vi "getSinglePathElement.vi"(8 "error in (no error)":errorcluster, 9 "Variant in":variant, 10 "JSON String":string, 11 "String":string) -> (0 "error out":errorcluster, 3 "Variant out":variant)   [LabVIEW 2015, in "Zen Analytics.lvclass"]
uses:
  Zen Analytics.lvclass
  <vilib>/addons/_JKI.lib/Serialization/JSON/JKI JSON Serialization.lvlib
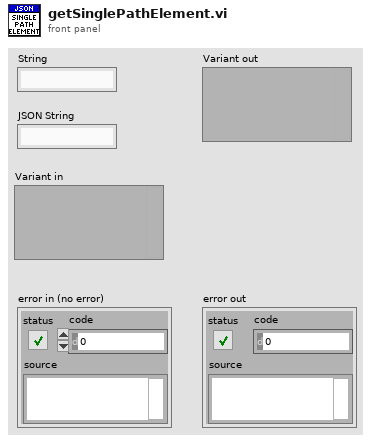
[diagram p1: front panel]
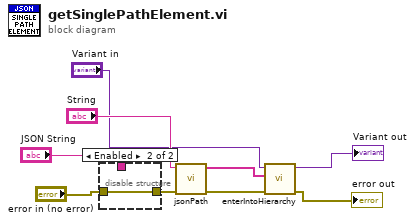
[diagram p0: block diagram]
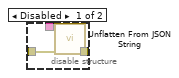
[diagram p2: hidden frame]
diagram:
  n1 = disable-structure shown="Enabled" {
    disable-tunnel: [w12 w13] -> w6
    disable-tunnel: "error in (no error)" -> [w11 w13]
    disable-tunnel: "JSON String" -> [w10 _]
    frame Disabled {
      n2 = call <vilib>:"Unflatten From JSON String.vi"("error in (no error)"=w11, "JSON String"=w10) -> ("error out"=w12:errorcluster)  [unwired: 8 in, 1 out]
    }
    frame Enabled {
    }
  }
  n3 = call "jsonPath.vi"("error in (no error)"=w6, "json path in"="String") -> ("error out"=w2:errorcluster, "output array of keys"=w7:string[])  [unwired: 8 in]
  n4 = call "enterIntoHierarchy.vi"("error in (no error)"=w2, "output array of keys"=w7, "Variant in"="Variant in") -> ("error out"=→"error out":errorcluster, "Variant out"=→"Variant out":variant)  [unwired: 7 in]
